vi "Check File Size.vi"(8 "error in (no error)":errorcluster, 11 "SQLite Database in":refnum<class "SQLite Database.lvclass">) -> (0 "error out":errorcluster, 3 "SQLite Database out":refnum<class "SQLite Database.lvclass">)   [LabVIEW 2019, in "TSC Event Logger.lvlib" / "SQLite Database.lvclass"]
uses:
  SQLite Database.lvclass
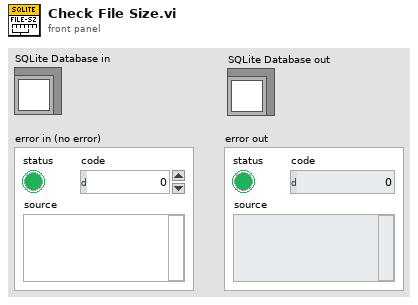
[diagram p1: front panel]
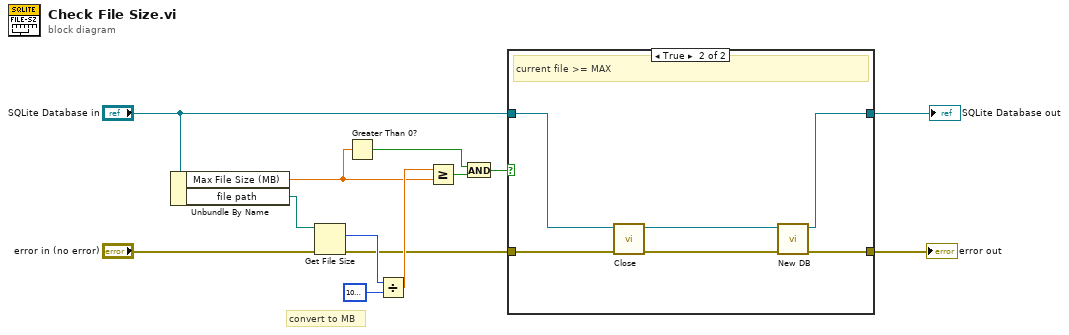
[diagram p0: block diagram]
diagram:
  # "convert to MB"
  n1 = Unbundle By Name("SQLite Database in") -> ("Max File Size (MB)"=w4:dbl, "file path"=w1:path)
  n2 = Get File Size(file=w1, error in="error in (no error)") -> (size (in bytes)=w11:i64, 0:w9:errorcluster)  [unwired: 1 out]
  n3 = Greater Than 0?(x=w4) -> (x > 0?=w2:bool)
  n4 = Divide(x=w11, y=i64 1000000) -> (x/y=w13:dbl)
  n5 = Greater Or Equal?(x=w13, y=w4) -> (x >= y?=w5:bool)
  n6 = And(x=w2, y=w5) -> (x .and. y?=w3:bool)
  n7 = case shown="True" w3 {
    tunnel: w9 -> [w14 w19]
    tunnel: "SQLite Database in" -> [w15 w18]
    tunnel: [w15 w20] -> w7
    tunnel: [w14 w21] -> w6
    frame False {
      # "file size fine, no change"
    }
    frame True {
      # "current file >= MAX"
      n8 = call-dynamic "Close.vi"("error in (no error)"=w19, "SQLite Database in"=w18) -> ("error out"=w17:errorcluster, "SQLite Database out"=w16:refnum<class "SQLite Database.lvclass">)  [unwired: 8 in]
      n9 = call "New DB.vi"("error in (no error)"=w17, "SQLite Database in"=w16) -> ("error out"=w21:errorcluster, "SQLite Database out"=w20:refnum<class "SQLite Database.lvclass">)  [unwired: 8 in]
    }
  }
  "error out" <- w6
  "SQLite Database out" <- w7
